vi "BOUCLE_YES_NO.vi"() -> (3 "OUI/NON":bool)   [LabVIEW 2020]
uses:
  VG_YESNON.vi
panel:
  out "errout":errorcluster caption="sortie d'erreur"
  in  "errin":errorcluster
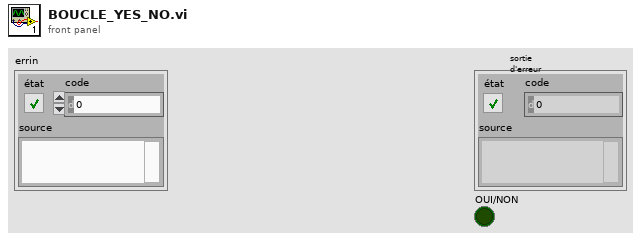
[diagram p1: front panel]
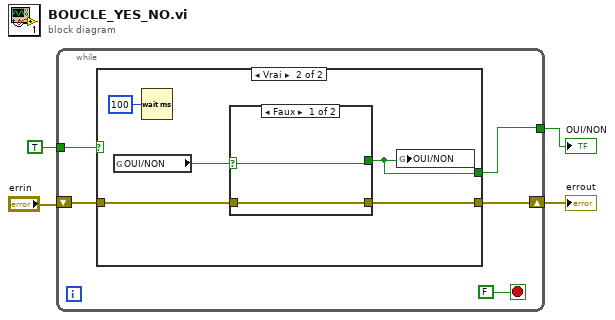
[diagram p0: block diagram]
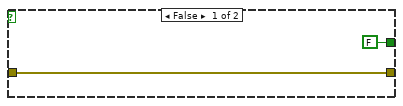
[diagram p2: hidden frame]
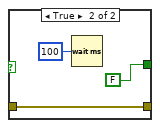
[diagram p3: hidden frame]
diagram:
  n1 = while {
    shift-right: [w8] -> w3
    shift-left: "errin" -> [w9]
    tunnel: [w6] -> w2
    tunnel: TRUE -> [w5]
    stop <- FALSE stop-if-true
    n2 = case shown="Vrai" w5 {
      tunnel: w9 -> [w11 w14]
      tunnel: [w11 w13] -> w8
      tunnel: [FALSE ("OUI/NON") w12] -> w6
      frame False {
      }
      frame True {
        n3 = global read "VG_YESNON.vi" "OUI/NON"() -> (w16:bool)
        n4 = Wait (ms)(milliseconds to wait=u32 100 ("attente (ms)")) -> ()  [unwired: 1 out]
        n5 = case shown="Faux" w16 {
          selector: w16 -> [w18 _]
          tunnel: [w18 FALSE ("OUI/NON")] -> w12
          tunnel: w14 -> [w17 w19]
          tunnel: [w17 w19] -> w13
          frame False {
          }
          frame True {
            n6 = Wait (ms)(milliseconds to wait=u32 100 ("attente (ms)")) -> ()  [unwired: 1 out]
          }
        }
        n7 = global write "VG_YESNON.vi" "OUI/NON"(w12) -> ()
      }
    }
  }
  "errout" <- w3
  "OUI/NON" <- w2
